vi "destroy buffer exchange.vi"(8 "error in":errorcluster, 9 "timeout in ms (0)":i32=200, 11 "exchange":T1) -> (0 "error out":errorcluster)   [LabVIEW 2013, in "tag bus buffer exchange.lvlib"]
uses:
  tag bus buffer exchange.lvlib
  buffer exchange.ctl
  buffer reference.ctl
  table/data table.ctl
  table/data table.lvlib
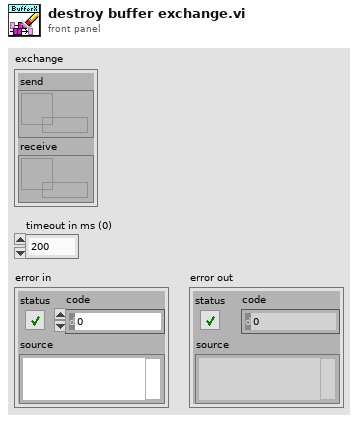
[diagram p1: front panel]
types:
  T1 = typedef "tag bus buffer exchange.lvlib/buffer exchange.ctl" = cluster{"send":refnum<k33>, "receive":refnum<k33>}
  T2 = typedef "tag bus buffer exchange.lvlib/buffer reference.ctl" = refnum<data-value>
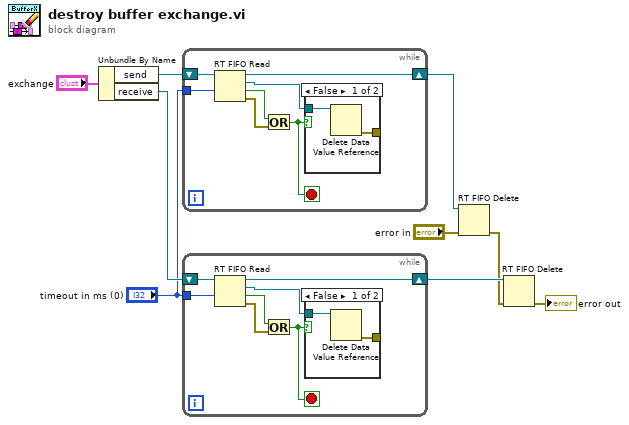
[diagram p0: block diagram]
diagram:
  n1 = Unbundle By Name("exchange") -> ("send"=w8:refnum<k33>, "receive"=w7:refnum<k33>)
  n2 = while {
    shift-right: [w15] -> w6
    shift-left: w8 -> [w16]
    tunnel: "timeout in ms (0)" -> [w10]
    stop <- w11 stop-if-true
    n3 = RT FIFO Read(0:w16, 2:w10) -> (8:w15:refnum<k33>, 9:w12:T2, 10:w14:bool, 11:w13:errorcluster)  [unwired: 2 in, 1 out]
    n4 = Or(x=w14, y=w13) -> (x .or. y?=w11:bool)
    n5 = case shown="False" w11 {
      tunnel: w12 -> [w18 _]
      tunnel: [w17 _] -> _
      frame False {
        n6 = Delete Data Value Reference(data value reference=w18) -> (error out=w17:errorcluster)  [unwired: 1 in, 1 out]
      }
      frame True {
      }
    }
  }
  n7 = while {
    shift-right: [w24] -> w5
    shift-left: w7 -> [w25]
    tunnel: "timeout in ms (0)" -> [w19]
    stop <- w20 stop-if-true
    n8 = RT FIFO Read(0:w25, 2:w19) -> (8:w24:refnum<k33>, 9:w21:T2, 10:w23:bool, 11:w22:errorcluster)  [unwired: 2 in, 1 out]
    n9 = Or(x=w23, y=w22) -> (x .or. y?=w20:bool)
    n10 = case shown="False" w20 {
      tunnel: w21 -> [w27 _]
      tunnel: [w26 _] -> _
      frame False {
        n11 = Delete Data Value Reference(data value reference=w27) -> (error out=w26:errorcluster)  [unwired: 1 in, 1 out]
      }
      frame True {
      }
    }
  }
  n12 = RT FIFO Delete(0:w6, 3:"error in") -> (11:w3:errorcluster)  [unwired: 1 in]
  n13 = RT FIFO Delete(0:w5, 3:w3) -> (11:→"error out":errorcluster)  [unwired: 1 in]
